vi "Run TS.vi"(8 "error in":errorcluster, 11 "Test Stand in":refnum<class "LNG Boiling Test Stand.lvclass">) -> (0 "error out":errorcluster, 3 "Test Stand out":refnum<class "LNG Boiling Test Stand.lvclass">)   [LabVIEW 2019, in "Test Stands.lvlib" / "LNG Boiling Test Stand.lvclass"]
uses:
  LNG Boiling Test Stand.lvclass
  DAC/DAC.lvclass
  Generic Test Stand/Generic Test Stand.lvclass
  Generic Test Stand/TS Panel Method.ctl
  C:/Users/wg/Documents/LV_Projects/test-stand/App/Generic Test Stand/Generic Test Stand.lvclass
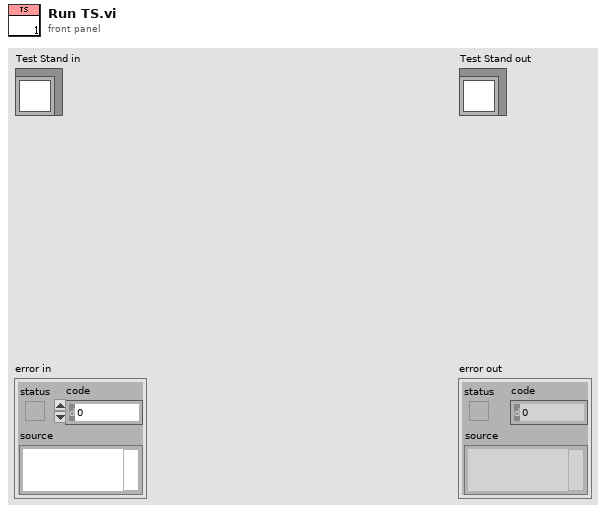
[diagram p1: front panel]
types:
  T1 = typedef "Generic Test Stand.lvclass/TS Panel Method.ctl" = enum16{"Send to Panel", "Receive from Panel"}
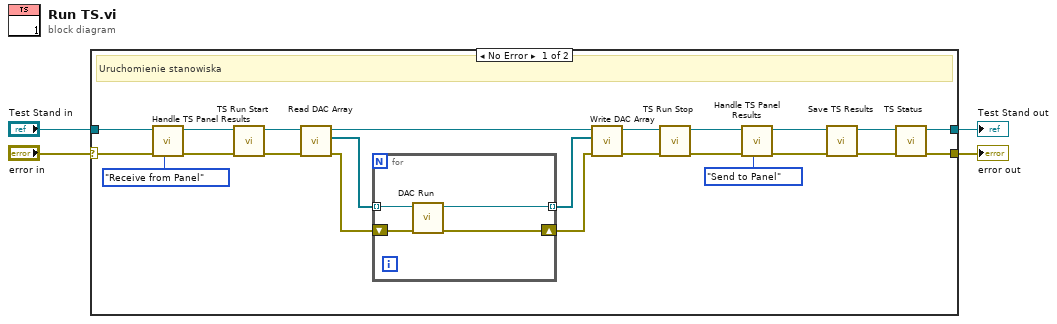
[diagram p0: block diagram]
diagram:
  n1 = case shown="No Error" "error in" {
    selector: "error in" -> [w13 w33]
    tunnel: "Test Stand in" -> [w14 w32]
    tunnel: [w6 w32] -> w1
    tunnel: [w5 w33] -> w4
    frame No Error {
      # "Uruchomienie stanowiska"
      n2 = call-dynamic "Handle TS Panel Results.vi"("Method"=TS_Panel_Method."Receive from Panel", "error in"=w13, "Test Stand in"=w14) -> ("error out"=w19:errorcluster, "Test Stand out"=w21:refnum<class "LNG Boiling Test Stand.lvclass">)  [unwired: 7 in]
      n3 = call-dynamic "TS Run Start.vi"("error in (no error)"=w19, "LNG Boiling Test Stand in"=w21) -> ("error out"=w10:errorcluster, "LNG Boiling Test Stand out"=w20:refnum<class "LNG Boiling Test Stand.lvclass">)  [unwired: 8 in]
      n4 = call "Read DAC Array.vi"("error in (no error)"=w10, "Generic Test Stand in"=w20) -> ("error out"=w9:errorcluster, "DAC Array"=w27:refnum<class "DAC.lvclass">[], "Generic Test Stand out"=w26:refnum<class "LNG Boiling Test Stand.lvclass">)  [unwired: 7 in]
      n5 = for {
        tunnel: w27 -> [w31] mode=indexing
        shift-right: [w28] -> w24
        shift-left: w9 -> [w30]
        tunnel: [w29] -> w25 mode=indexing
        n6 = call-dynamic "DAC Run.vi"("error in (no error)"=w30, "DAC in"=w31) -> ("error out"=w28:errorcluster, "DAC out"=w29:refnum<class "DAC.lvclass">)  [unwired: 8 in]
      }
      n7 = call "Write DAC Array.vi"("error in (no error)"=w24, "DAC Array"=w25, "Generic Test Stand in"=w26) -> ("error out"=w17:errorcluster, "Generic Test Stand out"=w18:refnum<class "LNG Boiling Test Stand.lvclass">)  [unwired: 7 in]
      n8 = call-dynamic "TS Run Stop.vi"("error in (no error)"=w17, "LNG Boiling Test Stand in"=w18) -> ("error out"=w15:errorcluster, "LNG Boiling Test Stand out"=w16:refnum<class "LNG Boiling Test Stand.lvclass">)  [unwired: 8 in]
      n9 = call-dynamic "Handle TS Panel Results.vi"("Method"=TS_Panel_Method."Send to Panel", "error in"=w15, "Test Stand in"=w16) -> ("error out"=w11:errorcluster, "Test Stand out"=w12:refnum<class "LNG Boiling Test Stand.lvclass">)  [unwired: 7 in]
      n10 = call-dynamic "Save TS Results.vi"("error in"=w11, "LNG Boiling Test Stand in"=w12) -> ("error out"=w7:errorcluster, "LNG Boiling Test Stand out"=w8:refnum<class "LNG Boiling Test Stand.lvclass">)  [unwired: 8 in]
      n11 = call-dynamic "TS Status.vi"("error in (no error)"=w7, "Generic Test Stand in"=w8) -> ("error out"=w5:errorcluster, "Generic Test Stand out"=w6:refnum<class "LNG Boiling Test Stand.lvclass">)  [unwired: 8 in]
    }
    frame Error {
    }
  }
  "error out" <- w4
  "Test Stand out" <- w1
